vi "Acquire Depth Image.vi"() -> ()   [LabVIEW 2014, in "LVH-KinectOne.lvlib"]
doc: "This example demonstrates how to acquire a depth frame from the Microsoft Kinect One."
uses:
  vi.lib/LabVIEW Hacker/KinectOne/LVH-KinectOne.lvlib
  vi.lib/LabVIEW Hacker/KinectOne/Private/kinectRead [DepthFrame].vi
panel:
  out "Depth Image":T1(plugin-control)
  in  "stop":bool
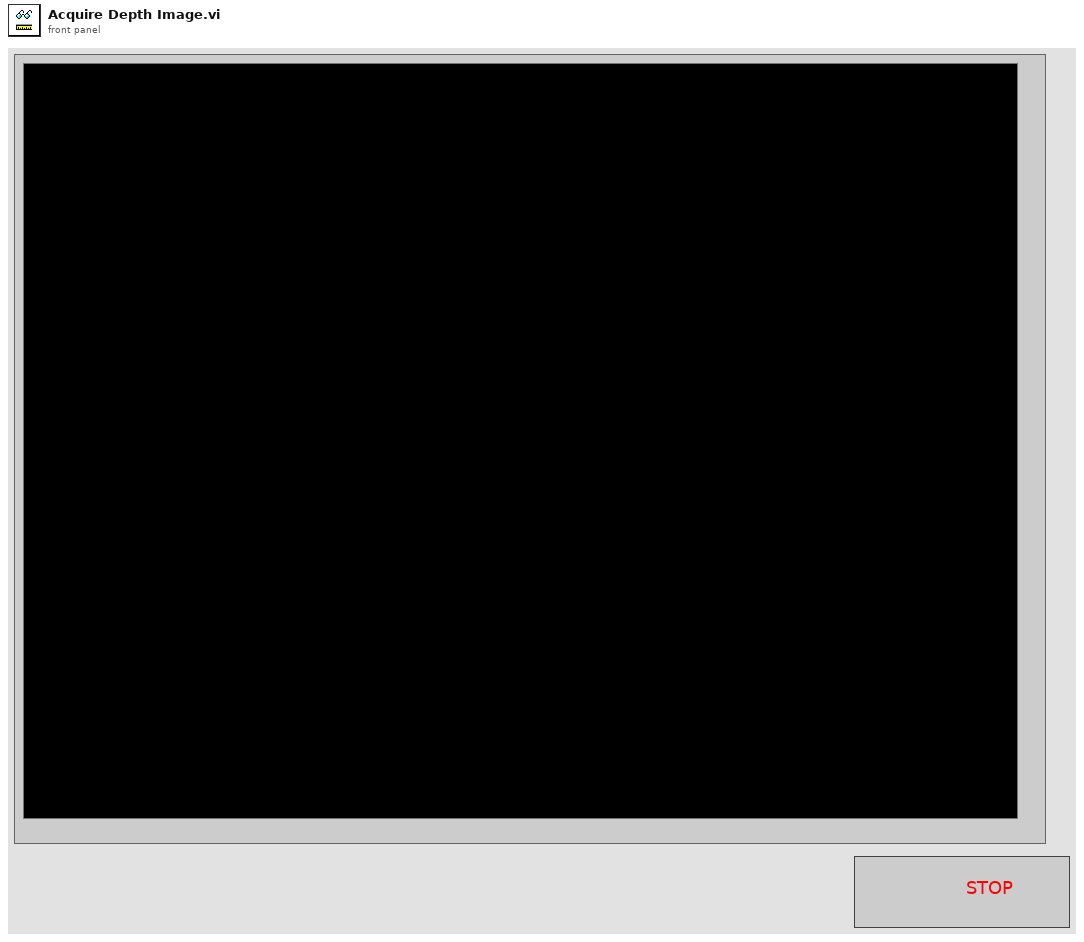
[diagram p1: front panel]
types:
  T1 = typedef "IMAQ Image.ctl" = refnum<image>
  T2 = typedef "Image Type" = u32
  T3 = typedef "LVH-KinectOne.lvlib/KinectSensor References.ctl" = cluster{"KinectSensor":refnum<k24>, "MultiSourceFrameReader":refnum<k24>, "BodyFrameDataInterface":refnum<k24>}
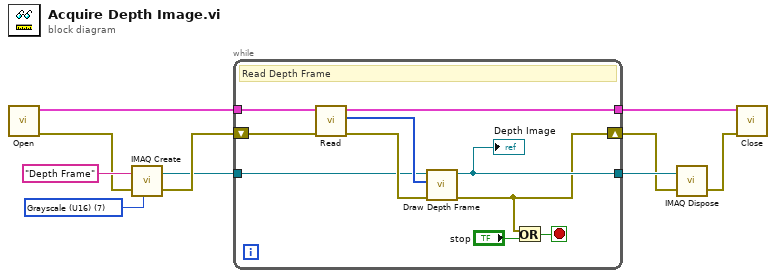
[diagram p0: block diagram]
diagram:
  w9 = T2 7 items=["Grayscale (U8)", "Grayscale (I16)", "Grayscale (SGL)", "Complex (CSG)", "RGB (U32)", "HSL (U32)", "RGB (U64)", "Grayscale (U16)"] ("Image Type")
  n1 = call "Open.vi"() -> ("error out"=w2:errorcluster, "KinectSensor References out"=w1:T3)  [unwired: 10 in]
  n2 = call "IMAQ Create"("Image Name"="Depth Frame", "Image Type"=w9, "error in (no error)"=w2) -> ("New Image"=w7:T1, "error out"=w8:errorcluster)  [unwired: 2 in]
  n3 = while {
    tunnel: w1 -> [w20]
    tunnel: [w16] -> w10
    shift-right: [w12] -> w5
    shift-left: w8 -> [w19]
    tunnel: w7 -> [w15]
    tunnel: [w14] -> w6
    stop <- w11 stop-if-true
    # "Read Depth Frame"
    n4 = call-poly "Read.vi"("error in (no error)"=w19, "KinectSensor References in"=w20) -> ("error out"=w18:errorcluster, "frameData"=w17:u16[], "KinectSensor References out"=w16:T3)  [unwired: 7 in]
    n5 = call "Draw Depth Frame.vi"("error in (no error)"=w18, "U16 Array"=w17, "Image"=w15) -> ("error out"=w12:errorcluster, "Image Out"=w14:T1)  [unwired: 7 in]
    "Depth Image" <- w14
    n6 = Or(x=w12, y="stop") -> (x .or. y?=w11:bool)
  }
  n7 = call "IMAQ Dispose"("Image"=w6, "error in (no error)"=w5) -> ("error out"=w4:errorcluster)  [unwired: 4 in]
  n8 = call "Close.vi"("error in"=w4, "KinectSensor References"=w10) -> ()  [unwired: 9 in, 1 out]
